vi "Get Sheet.vi"(8 "error in":errorcluster, 10 "SheetName":string, 11 "SpreadsheetDoc in":refnum<k24>) -> (0 "error out":errorcluster, 1 "Sheet Index":i32, 2 "Sheet":refnum<k24>, 3 "SpreadsheetDoc out":refnum<k24>, 5 "SheetName":string)   [LabVIEW 2019, in "Open Xml.lvlib"]
doc: "Returns first sheet on empty Sheet Name"
uses:
  Open Xml.lvlib
  D:/git/Open-Xml-LabVIEW/Source/DocumentFormat.OpenXml.dll
  DocumentFormat.OpenXml.dll
  D:/git/Open-Xml-LabVIEW/Source/DocumentFormat.OpenXml.Framework.dll
  DocumentFormat.OpenXml.Framework.dll
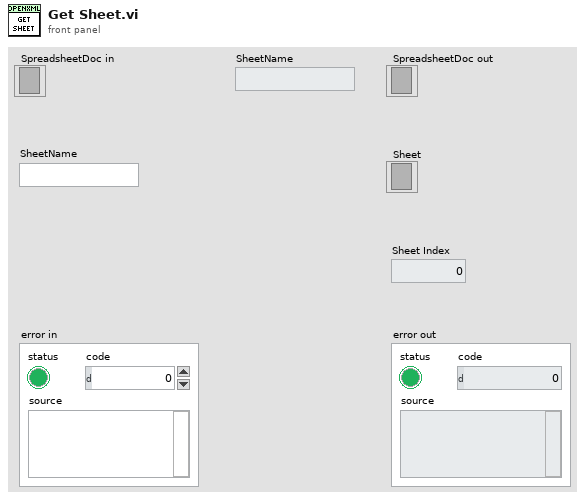
[diagram p1: front panel]
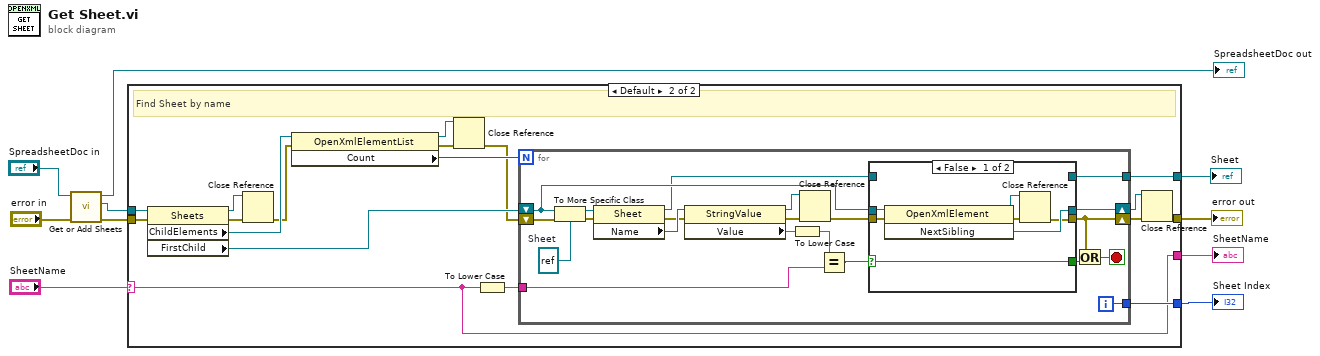
[diagram p0: block diagram]
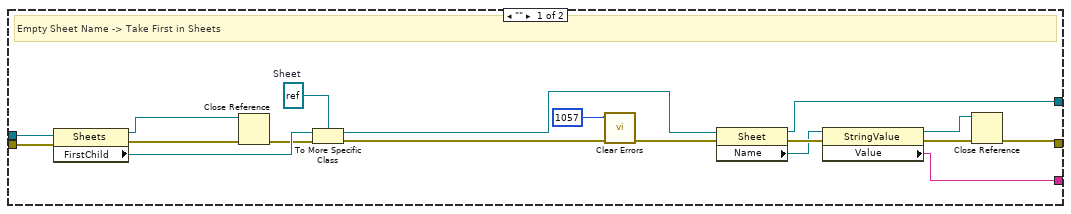
[diagram p2: hidden frame]
diagram:
  n1 = call "Get or Add Sheets.vi"("error in"="error in", "SpreadsheetDoc in"="SpreadsheetDoc in") -> ("error out"=w7:errorcluster, "Sheets"=w8:refnum<k24>, "SpreadsheetDoc out"=→"SpreadsheetDoc out":refnum<k24>)  [unwired: 7 in]
  n2 = case shown="Default" "SheetName" {
    selector: "SheetName" -> [_ w30]
    tunnel: w8 -> [w27 w42]
    tunnel: w7 -> [w28 w41]
    tunnel: [w16 w39] -> w4
    tunnel: [w12 w37] -> w3
    tunnel: [_ w31] -> w2
    tunnel: [w13 w30] -> w1
    frame "" {
      w25 = refnum<k24> refnum  # Sheet
      # "Empty Sheet Name -> Take First in Sheets"
      n3 = property class="Sheets"(reference=w27, error in=w28) -> (reference out=w22:refnum<k24>, error out=w26:errorcluster, "FirstChild"=w24:refnum<k24>)
      n4 = Close Reference(reference=w22, error in (no error)=w26) -> (error out=w23:errorcluster)
      n5 = To More Specific Class(target class=w25, reference=w24, error in=w23) -> (specific class reference=w17:refnum<k24>, error out=w21:errorcluster)
      n6 = call <vilib>:"Clear Errors.vi"("error in (no error)"=w21, "specific error code to clear (0: all)"=1057) -> ("error out"=w20:errorcluster)  [unwired: 4 in, 1 out]
      n7 = property class="Sheet"(reference=w17, error in=w20) -> (reference out=w16:refnum<k24>, error out=w18:errorcluster, "Name"=w14:refnum<k24>)
      n8 = property class="StringValue"(reference=w14, error in=w18) -> (reference out=w11:refnum<k24>, error out=w15:errorcluster, "Value"=w13:string)
      n9 = Close Reference(reference=w11, error in (no error)=w15) -> (error out=w12:errorcluster)
    }
    frame Default {
      # "Find Sheet by name"
      n10 = property class="Sheets"(reference=w42, error in=w41) -> (reference out=w40:refnum<k24>, error out=w46:errorcluster, "ChildElements"=w44:refnum<k24>, "FirstChild"=w45:refnum<k24>)
      n11 = Close Reference(reference=w40, error in (no error)=w46) -> (error out=w35:errorcluster)
      n12 = property class="OpenXmlElementList"(reference=w44, error in=w35) -> (reference out=w32:refnum<k24>, error out=w34:errorcluster, "Count"=w43:i32)
      n13 = Close Reference(reference=w32, error in (no error)=w34) -> (error out=w33:errorcluster)
      n14 = To Lower Case(string=w30) -> (all lower case string=w29:string)
      n15 = for {
        N: w43 -> [_]
        shift-right: [w60] -> w36
        shift-left: w45 -> [w63]
        tunnel: w29 -> [w61]
        tunnel: [w54] -> w39
        shift-right: [w55] -> w38
        shift-left: w33 -> [w66]
        tunnel: [w48] -> w31
        i -> [w48]
        stop <- w56 stop-if-true
        w67 = refnum<k24> refnum  # Sheet
        n16 = To More Specific Class(target class=w67, reference=w63, error in=w66) -> (specific class reference=w62:refnum<k24>, error out=w65:errorcluster)
        n17 = property class="Sheet"(reference=w62, error in=w65) -> (reference out=w59:refnum<k24>, error out=w51:errorcluster, "Name"=w53:refnum<k24>)
        n18 = property class="StringValue"(reference=w53, error in=w51) -> (reference out=w49:refnum<k24>, error out=w50:errorcluster, "Value"=w52:string)
        n19 = To Lower Case(string=w52) -> (all lower case string=w47:string)
        n20 = Close Reference(reference=w49, error in (no error)=w50) -> (error out=w64:errorcluster)
        n21 = Equal?(x=w47, y=w61) -> (x = y?=w58:bool)
        n22 = case shown="False" w58 {
          selector: w58 -> [w71 w77]
          tunnel: w64 -> [w74 w76]
          tunnel: [w68 w76] -> w55
          tunnel: w63 -> [w73 _]
          tunnel: [w72 _] -> w60
          tunnel: w59 -> [_ w75]
          tunnel: [w71 w77] -> w57
          tunnel: [_ w75] -> w54
          frame False {
            n23 = invoke class="OpenXmlElement" method="NextSibling"(reference=w73, error in=w74) -> (reference out=w70:refnum<k24>, error out=w69:errorcluster, "NextSibling"=w72:refnum<k24>)  [unwired: 1 in]
            n24 = Close Reference(reference=w70, error in (no error)=w69) -> (error out=w68:errorcluster)
          }
          frame True {
          }
        }
        n25 = Or(x=w55, y=w57) -> (x .or. y?=w56:bool)
      }
      n26 = Close Reference(reference=w36, error in (no error)=w38) -> (error out=w37:errorcluster)
    }
  }
  "error out" <- w3
  "Sheet" <- w4
  "Sheet Index" <- w2
  "SheetName" <- w1
